vi "Drive Towards Gap.vi"(6 "max angular velocity (rad/s)":dbl=1.0, 7 "max reverse velocity (m/s)":dbl, 8 "error in (no error)":errorcluster, 10 "findA":bool, 11 "angle":dbl) -> (0 "error out":errorcluster, 3 "steering frame velocity":dbl[](array[numeric]))   [LabVIEW 2012]
doc: "Sets the steering frame velocity so that the robot moves towards the gap."
uses:
  <vilib>/robotics/Obstacle Avoidance/Simple Vector Field Histogram/Gap Description.ctl
  <vilib>/robotics/Obstacle Avoidance/Simple Vector Field Histogram/NI_Robotics_Simple Vector Field Histogram.lvlib
panel:
  in  "gap":T1
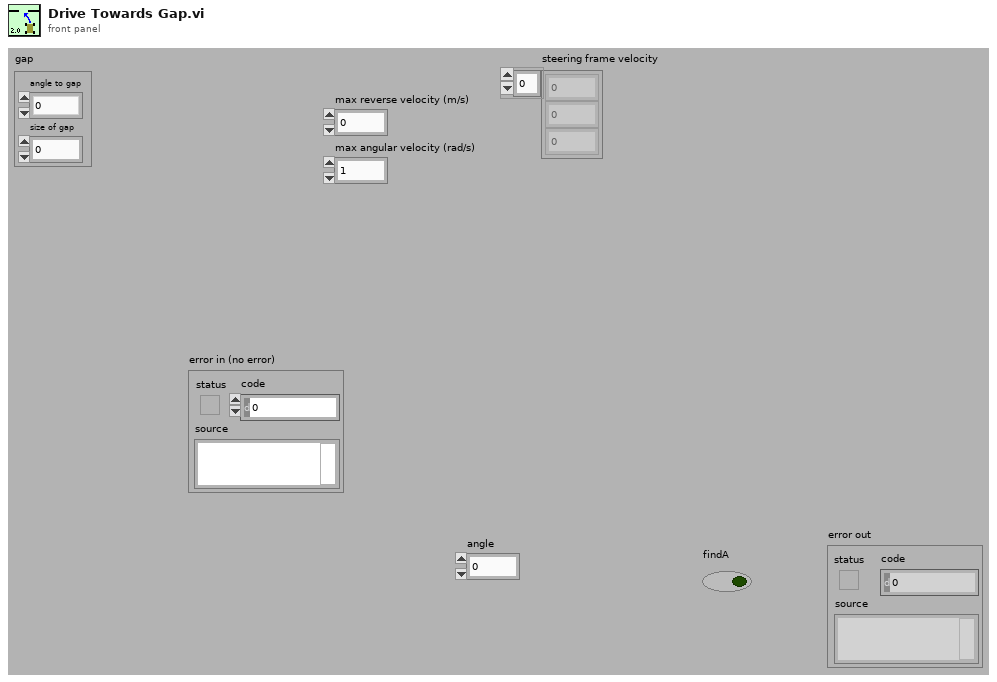
[diagram p1: front panel]
types:
  T1 = typedef "NI_Robotics_Simple Vector Field Histogram.lvlib/Gap Description.ctl" = cluster{"angle to gap":dbl, "size of gap":dbl}
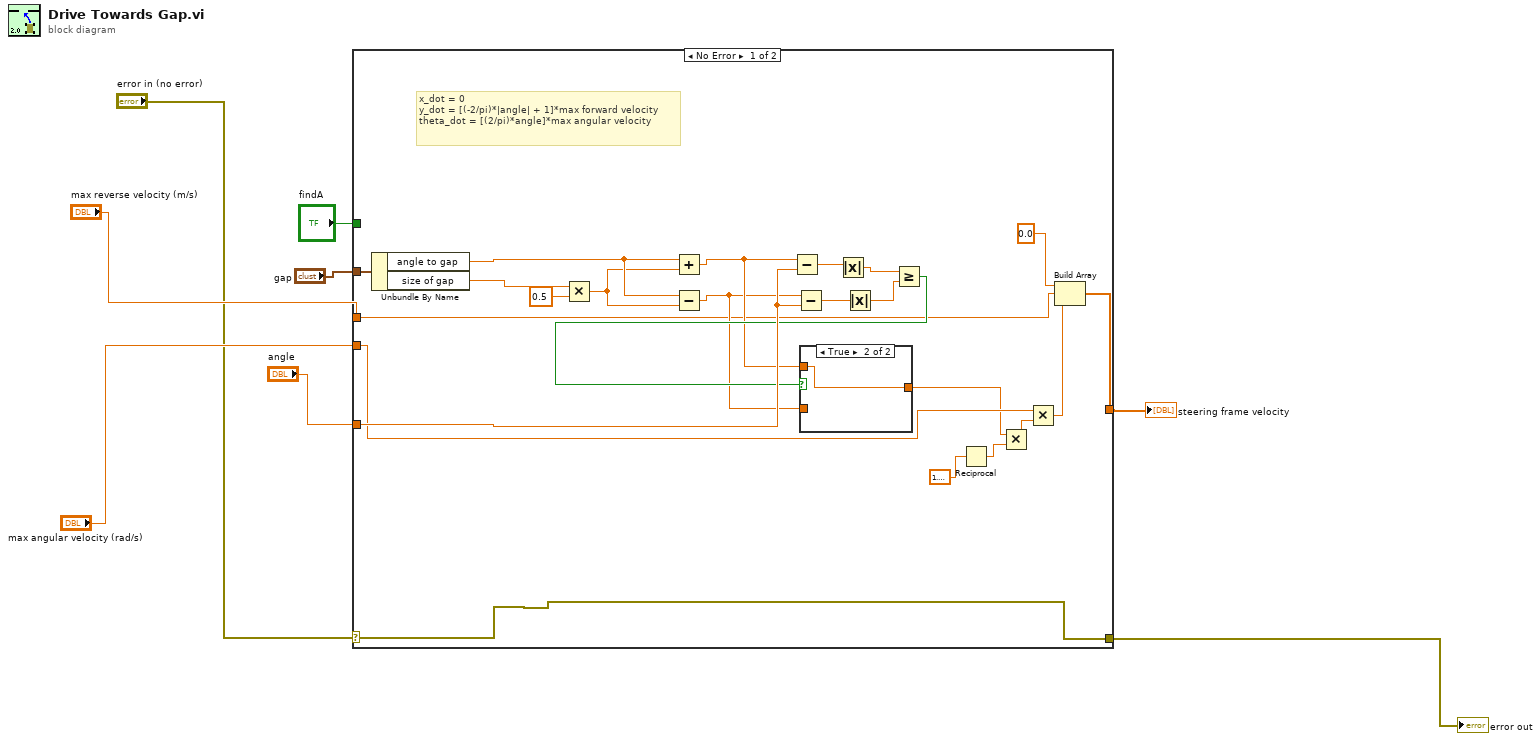
[diagram p0: block diagram]
diagram:
  n1 = case shown="No Error" "error in (no error)" {
    selector: "error in (no error)" -> [w30 w34]
    tunnel: [w30 w34] -> w4
    tunnel: "max reverse velocity (m/s)" -> [w13 _]
    tunnel: "angle" -> [w31 _]
    tunnel: "max angular velocity (rad/s)" -> [w11 _]
    tunnel: "gap" -> [w29 _]
    tunnel: [w28 _] -> w2
    tunnel: "findA" -> [_ _]
    frame No Error {
      # "x_dot = 0\ny_dot = [(-2/pi)*|angle| + 1]*max forward velocity\ntheta_dot = [(2/pi)*angle]*max angular velocity"
      n2 = Unbundle By Name(w29) -> ("angle to gap"=w27:dbl, "size of gap"=w26:dbl)
      n3 = Multiply(x=w26, y=0.5) -> (x*y=w24:dbl)
      n4 = Add(x=w27, y=w24) -> (x+y=w18:dbl)
      n5 = Subtract(x=w27, y=w24) -> (x-y=w17:dbl)
      n6 = Subtract(x=w18, y=w31) -> (x-y=w23:dbl)
      n7 = Subtract(x=w17, y=w31) -> (x-y=w22:dbl)
      n8 = Absolute Value(x=w23) -> (abs(x)=w21:dbl)
      n9 = Absolute Value(x=w22) -> (abs(x)=w20:dbl)
      n10 = Greater Or Equal?(x=w21, y=w20) -> (x >= y?=w19:bool)
      n11 = case shown="True" w19 {
        tunnel: w18 -> [_ w33]
        tunnel: w17 -> [w32 _]
        tunnel: [w32 w33] -> w9
        frame False {
        }
        frame True {
        }
      }
      n12 = Reciprocal(x=1.5707963267948966) -> (1/x=w14:dbl)
      n13 = Multiply(x=w9, y=w14) -> (x*y=w10:dbl)
      n14 = Multiply(x=w11, y=w10) -> (x*y=w12:dbl)
      n15 = Build Array(0.0 ("element"), w13, w12) -> (w28:dbl[])
    }
    frame Error {
    }
  }
  "error out" <- w4
  "steering frame velocity" <- w2
